vi "Test_SI656vi.vi"(5 "start Datetime":cluster{"row":i32, "column":i32}={"row"=1, "column"=0}, 7 "end Datetime":cluster{"row":i32, "column":i32}={"row"=3504, "column"=0}, 9 "start Data":cluster{"start row":i32, "start column":i32}={"start row"=1, "start column"=1}, 11 "end Data":cluster{"row":i32, "column":i32}={"row"=3504, "column"=4}) -> (6 "Measurements":cluster{timestamp[], dbl[][]}, 8 "XY Graph":cluster{timestamp[], dbl[]}[](graph))   [LabVIEW 2022 SP3]
uses:
  <vilib>/Utility/NIReport.llb/Report Type.ctl
  <vilib>/addons/_office/excel.llb/Excel Get Data ([str]).vi
  <vilib>/addons/_office/excel.llb/Excel Get Data ([dbl]).vi
  <vilib>/Utility/NIReport.llb/NI_report.lvclass
  <vilib>/addons/_office/NI_ReportGenerationToolkit.lvlib
  <vilib>/Utility/NIReport.llb/NI_ReportGenerationCore.lvlib
  <vilib>/Utility/NIReport.llb/Excel/NI_Excel.lvclass
panel:
  out "time stamp":timestamp[](array[timestamp])
  out "Date":string[][](array[string])
  out "data":dbl[][](array[numeric]) format="%.2f"
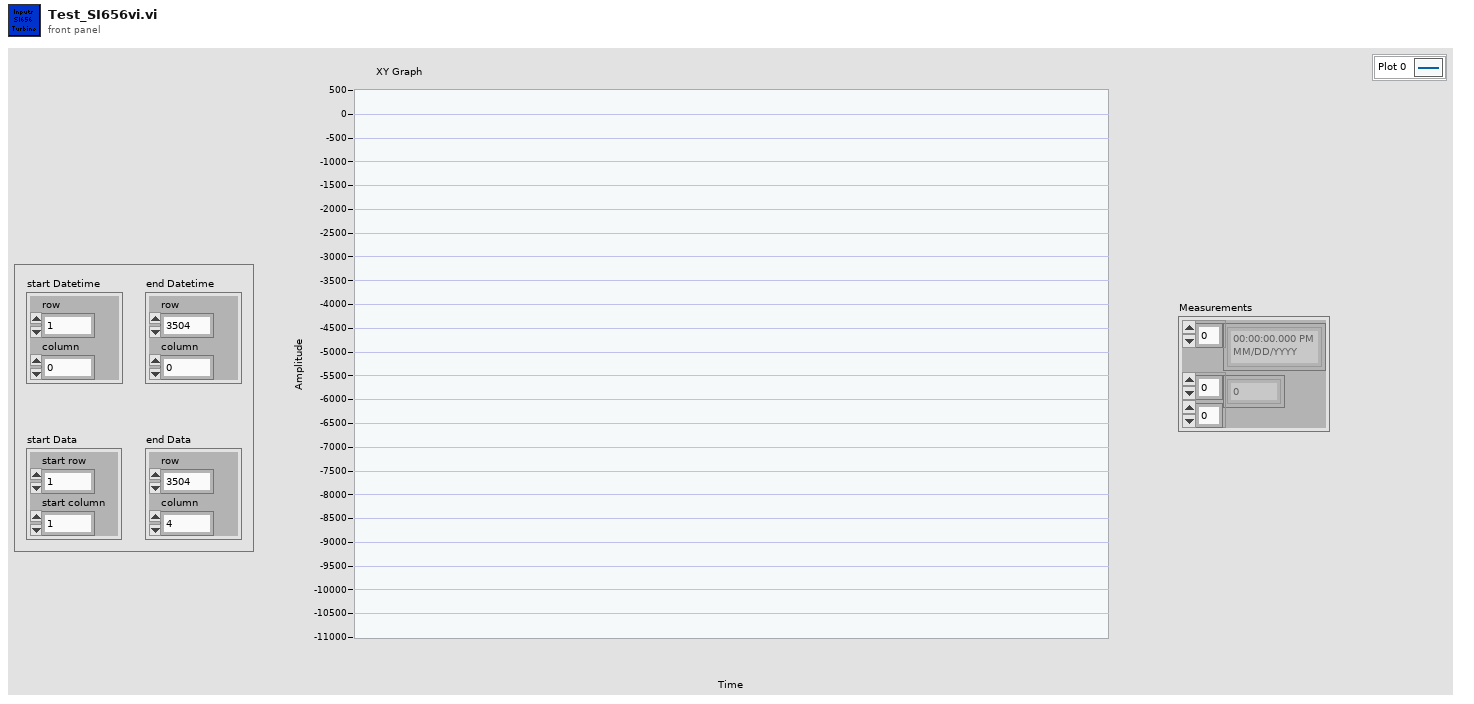
[diagram p1: front panel]
types:
  T1 = typedef "NI_ReportGenerationCore.lvlib/Report Type.ctl" = enum16{"HTML", "Word", "Excel"}
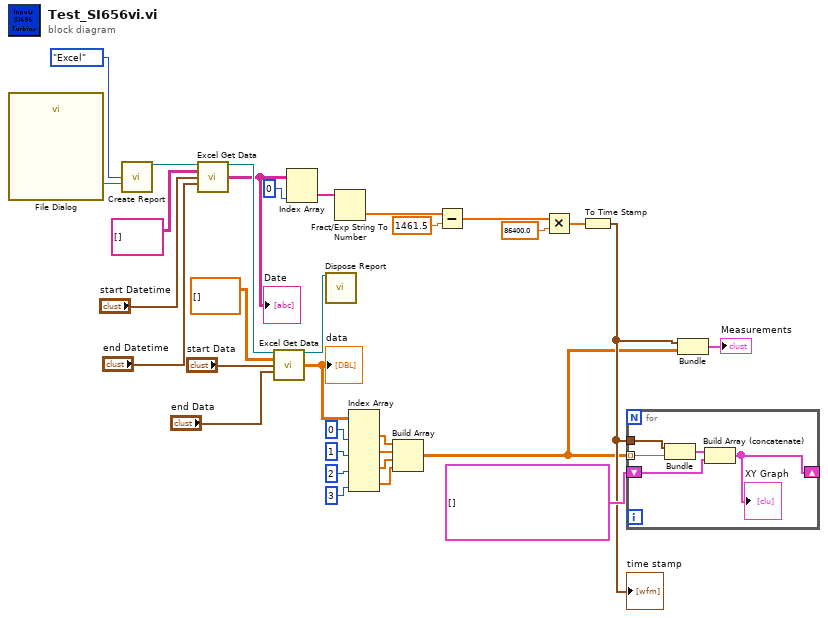
[diagram p0: block diagram]
diagram:
  n1 = call "File Dialog"() -> ("selected path"=w27:path)  [unwired: 12 in, 3 out]
  n2 = call <vilib>:"Create Report.vi"("report type"=Report_Type."Excel", "template (empty)"=w27) -> ("report out"=w26:refnum<class "NI_report.lvclass">)  [unwired: 12 in, 1 out]
  n3 = call-poly <vilib>:"Excel Get Data.vi"("report in"=w26, "data type"=string[][] [], "start (-1, -1)"="start Datetime", "end (-1, -1)"="end Datetime") -> ("report out"=w22:refnum<class "NI_report.lvclass">, "data"=w8:string[][])  [unwired: 9 in, 1 out]
  "Date" <- w8
  n4 = call-poly <vilib>:"Excel Get Data.vi"("report in"=w22, "data type"=dbl[][] [], "start (-1, -1)"="start Data", "end (-1, -1)"="end Data") -> ("report out"=w29:refnum<class "NI_report.lvclass">, "data"=w17:dbl[][])  [unwired: 9 in, 1 out]
  "data" <- w17
  n5 = Index Array(array=w8, index (col)=0 ("disabled index (col)")) -> (element=w6:string[])  [unwired: 1 in]
  n6 = call-dynamic "Dispose Report.vi"("report in"=w29) -> ()  [unwired: 14 in, 1 out]
  n7 = Fract/Exp String To Number(string=w6) -> (number=w13:dbl[])  [unwired: 3 in, 1 out]
  n8 = Index Array(array=w17, index (col) #1=0 ("disabled index (col)"), index (col) #2=1 ("index (col)"), index (col) #3=2 ("index (col)"), index (col) #4=3 ("index (col)")) -> (element #1=w5:dbl[], element #2=w16:dbl[], element #3=w15:dbl[], element #4=w14:dbl[])  [unwired: 4 in]
  n9 = Build Array(w5, w16, w15, w14) -> (w2:dbl[][])
  n10 = Subtract(x=w13, y=1461.5) -> (x-y=w11:dbl[])
  n11 = Multiply(x=w11, y=86400.0) -> (x*y=w9:dbl[])
  n12 = To Time Stamp(1:w9) -> (0:w3:timestamp[])
  "time stamp" <- w3
  n13 = for {
    tunnel: w2 -> [w37] mode=indexing
    tunnel: w3 -> [w36]
    shift-right: [w34] -> _
    shift-left: cluster{timestamp[], dbl[]}[] [] -> [w33]
    n14 = Bundle(w36, w37) -> (w35:cluster{timestamp[], dbl[]})  [unwired: 1 in]
    n15 = Build Array (concatenate)(w35, w33) -> (w34:cluster{timestamp[], dbl[]}[])
    "XY Graph" <- w34
  }
  n16 = Bundle(w3, w2) -> (→"Measurements":cluster{timestamp[], dbl[][]})  [unwired: 1 in]
